vi "Set Security Level CORE.vi"(8 "error in (no error)":errorcluster, 9 "Set or Clear":T1, 10 "Security Level":T2, 11 "Threat Deterents in":refnum<class "Threat Deterents.lvclass">) -> (0 "error out":errorcluster, 2 "Last Action Performed":string, 3 "Threat Deterents out":refnum<class "Threat Deterents.lvclass">)   [LabVIEW 2020, in "Threat Deterents.lvclass"]
uses:
  Threat Deterents.lvclass
  Security System/Security Level.ctl
  Security System/Set or Clear.ctl
  Threat Deterents.lvclass/Threat Deterents.ctl
  Electric Fences/Electric Fences.lvclass
  Security System/Security System.lvclass
  Rabbit Squad/Rabbit Squad.lvclass
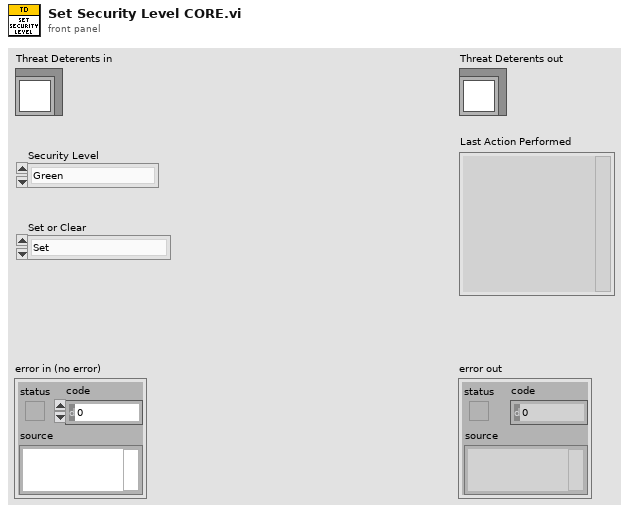
[diagram p1: front panel]
types:
  T1 = typedef "Security System.lvclass/Set or Clear.ctl" = enum16{"Set", "Clear"}
  T2 = typedef "Security System.lvclass/Security Level.ctl" = enum16{"Green", "Yellow", "Orange", "Red"}
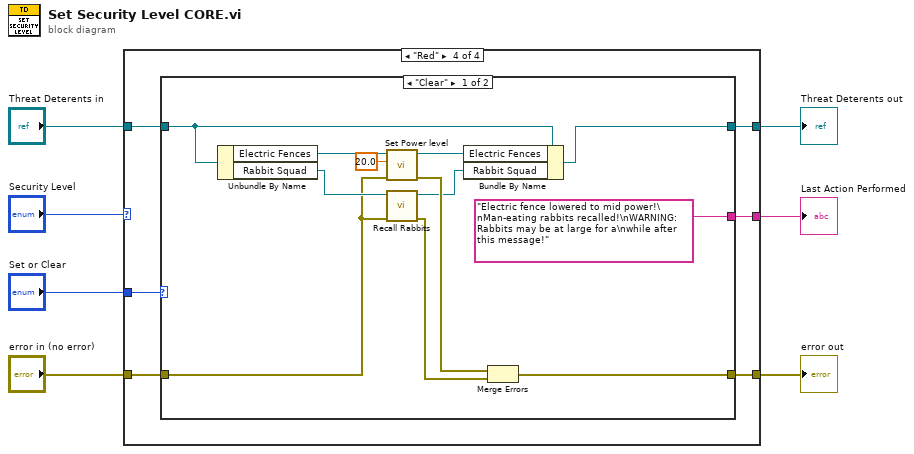
[diagram p0: block diagram]
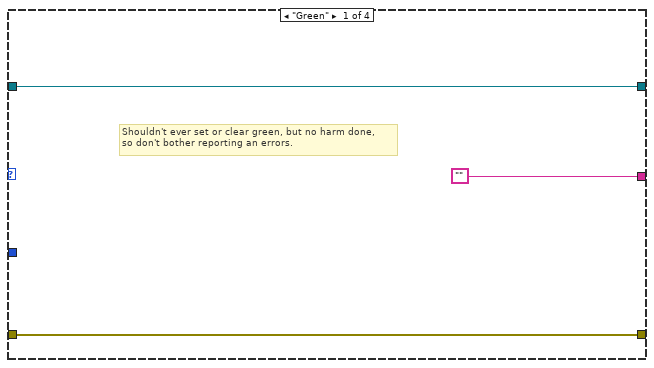
[diagram p2: hidden frame]
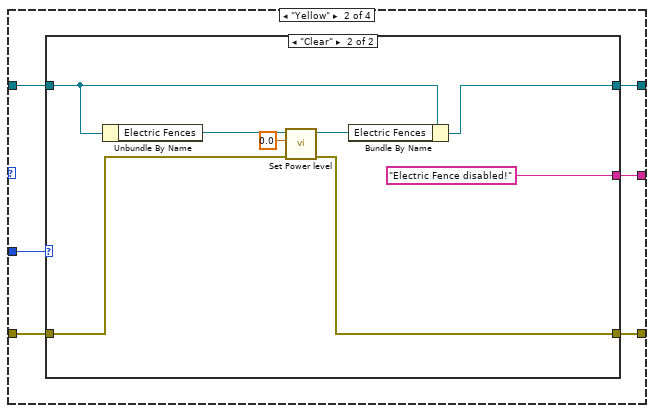
[diagram p3: hidden frame]
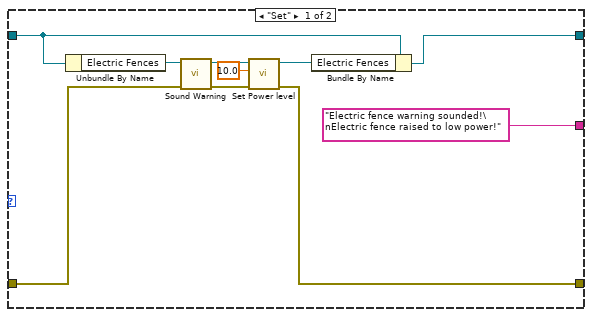
[diagram p4: hidden frame]
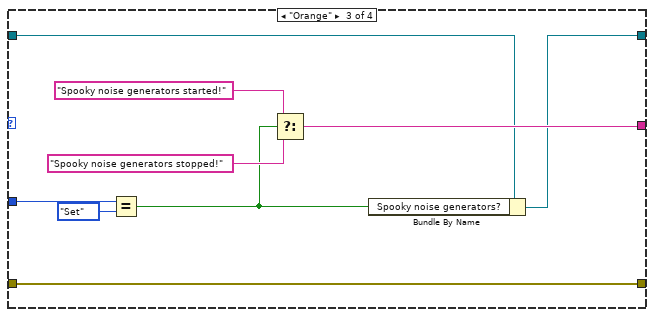
[diagram p5: hidden frame]
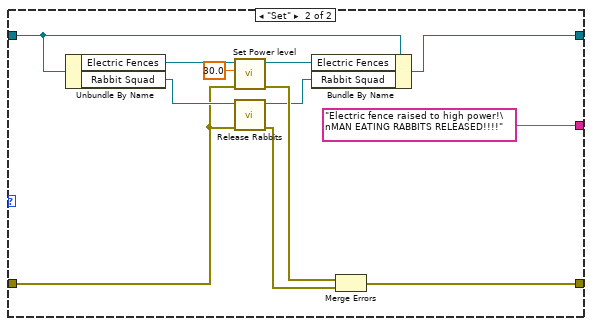
[diagram p6: hidden frame]
diagram:
  n1 = case shown="\"Red\"" "Security Level" {
    tunnel: "Set or Clear" -> [_ w16 w42 w49]
    tunnel: "error in (no error)" -> [w9 w13 w43 w46]
    tunnel: [w9 w12 w43 w45] -> w5
    tunnel: "Threat Deterents in" -> [w10 w15 w37 w48]
    tunnel: [w10 w14 w36 w47] -> w2
    tunnel: ["" w11 w38 w44] -> w1
    frame "Green" {
      # "Shouldn't ever set or clear green, but no harm done,\nso don't bother reporting an errors."
    }
    frame "Yellow" {
      n2 = case shown="\"Clear\"" w16 {
        tunnel: w15 -> [w20 w32]
        tunnel: [w18 w30] -> w14
        tunnel: w13 -> [w25 w27]
        tunnel: [w22 w34] -> w12
        tunnel: ["Electric fence warning sounded!\nElectric fence raised to low power!" "Electric Fence disabled!"] -> w11
        frame "Set" {
          n3 = Unbundle By Name(w20) -> ("Electric Fences"=w26:refnum<class "Electric Fences.lvclass">)
          n4 = call "Sound Warning.vi"("error in (no error)"=w25, "Electric Fences in"=w26) -> ("error out"=w23:errorcluster, "Electric Fences out"=w24:refnum<class "Electric Fences.lvclass">)  [unwired: 8 in]
          n5 = call-dynamic "Set Power level"("error in (no error)"=w23, "Power level"=10.0, "Electric Fences in"=w24) -> ("error out"=w22:errorcluster, "Electric Fences out"=w19:refnum<class "Electric Fences.lvclass">)  [unwired: 7 in]
          n6 = Bundle By Name(cluster=w20, "Electric Fences"=w19) -> (w18:refnum<class "Threat Deterents.lvclass">)
        }
        frame "Clear" {
          n7 = Unbundle By Name(w32) -> ("Electric Fences"=w28:refnum<class "Electric Fences.lvclass">)
          n8 = call-dynamic "Set Power level"("error in (no error)"=w27, "Power level"=0.0, "Electric Fences in"=w28) -> ("error out"=w34:errorcluster, "Electric Fences out"=w31:refnum<class "Electric Fences.lvclass">)  [unwired: 7 in]
          n9 = Bundle By Name(cluster=w32, "Electric Fences"=w31) -> (w30:refnum<class "Threat Deterents.lvclass">)
        }
      }
    }
    frame "Orange" {
      n10 = Equal?(x=w42, y=Set_or_Clear."Set") -> (x = y?=w35:bool)
      n11 = Select(t="Spooky noise generators started!", s=w35, f="Spooky noise generators stopped!") -> (s? t:f=w38:string)
      n12 = Bundle By Name(cluster=w37, "Spooky noise generators?"=w35) -> (w36:refnum<class "Threat Deterents.lvclass">)
    }
    frame "Red" {
      n13 = case shown="\"Clear\"" w49 {
        tunnel: w48 -> [w60 w72]
        tunnel: [w58 w70] -> w47
        tunnel: w46 -> [w51 w63]
        tunnel: [w54 w66] -> w45
        tunnel: ["Electric fence lowered to mid power!\nMan-eating rabbits recalled!\nWARNING: Rabbits may be at large for a\nwhile after this message!" "Electric fence raised to high power!\nMAN EATING RABBITS RELEASED!!!!"] -> w44
        frame "Clear" {
          n14 = Unbundle By Name(w60) -> ("Electric Fences"=w56:refnum<class "Electric Fences.lvclass">, "Rabbit Squad"=w53:refnum<class "Rabbit Squad.lvclass">)
          n15 = call-dynamic "Set Power level"("error in (no error)"=w51, "Power level"=20.0, "Electric Fences in"=w56) -> ("error out"=w55:errorcluster, "Electric Fences out"=w59:refnum<class "Electric Fences.lvclass">)  [unwired: 7 in]
          n16 = call "Recall Rabbits.vi"("error in (no error)"=w51, "Rabbit Squad in"=w53) -> ("error out"=w50:errorcluster, "Rabbit Squad out"=w52:refnum<class "Rabbit Squad.lvclass">)  [unwired: 8 in]
          n17 = Bundle By Name(cluster=w60, "Electric Fences"=w59, "Rabbit Squad"=w52) -> (w58:refnum<class "Threat Deterents.lvclass">)
          n18 = Merge Errors(w55, w50) -> (w54:errorcluster)
        }
        frame "Set" {
          n19 = Unbundle By Name(w72) -> ("Electric Fences"=w68:refnum<class "Electric Fences.lvclass">, "Rabbit Squad"=w65:refnum<class "Rabbit Squad.lvclass">)
          n20 = call-dynamic "Set Power level"("error in (no error)"=w63, "Power level"=30.0, "Electric Fences in"=w68) -> ("error out"=w67:errorcluster, "Electric Fences out"=w71:refnum<class "Electric Fences.lvclass">)  [unwired: 7 in]
          n21 = call "Release Rabbits.vi"("error in (no error)"=w63, "Rabbit Squad in"=w65) -> ("error out"=w62:errorcluster, "Rabbit Squad out"=w64:refnum<class "Rabbit Squad.lvclass">)  [unwired: 8 in]
          n22 = Bundle By Name(cluster=w72, "Electric Fences"=w71, "Rabbit Squad"=w64) -> (w70:refnum<class "Threat Deterents.lvclass">)
          n23 = Merge Errors(w67, w62) -> (w66:errorcluster)
        }
      }
    }
  }
  "error out" <- w5
  "Threat Deterents out" <- w2
  "Last Action Performed" <- w1
